vi "Get Subsystem Names.vi"(8 "error in (no error)":errorcluster, 11 "Server URL":refnum<k21>) -> (0 "error out":errorcluster, 2 "Subsystem Names":string[](array[string]), 3 "dup Server URL":refnum<k21>)   [LabVIEW 2024]
doc: "Gets the subsystem names."
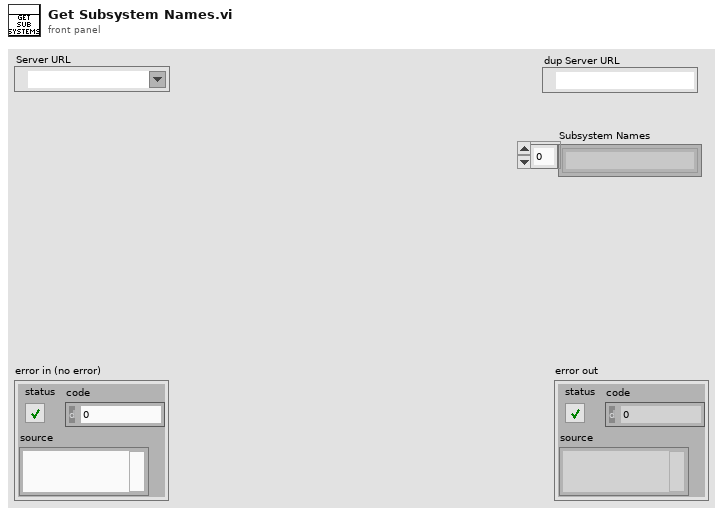
[diagram p1: front panel]
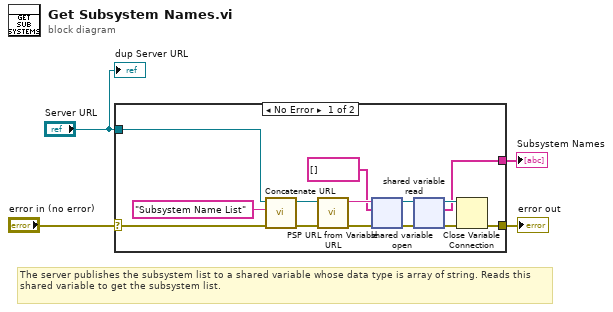
[diagram p0: block diagram]
diagram:
  # "The server publishes the subsystem list to a shared variable whose data type is array of string. Reads this shared variable to get the subsystem list."
  n1 = case shown="No Error" "error in (no error)" {
    selector: "error in (no error)" -> [w18 w19]
    tunnel: [w5 w19] -> w3
    tunnel: "Server URL" -> [w8 _]
    tunnel: [w6 _] -> w1
    frame No Error {
      n2 = call "Concatenate URL.vi"("error in (no error)"=w18, "Child Name"="Subsystem Name List", "Parent URL"=w8) -> ("error out"=w17:errorcluster, "Child URL"=w14:refnum<k21>)  [unwired: 7 in]
      n3 = call "PSP URL from Variable URL.vi"("error in (no error)"=w17, "Shared Variable URL"=w14) -> ("error out"=w16:errorcluster, "PSP URL"=w15:string)  [unwired: 8 in]
      n4 = shared-variable-open(w15, w16, string[] []) -> (w11:refnum<k21>, w12:errorcluster)  [unwired: 1 in]
      n5 = shared-variable-read(w11, w12) -> (w9:refnum<k21>, w10:errorcluster, w6:string[])  [unwired: 1 out]
      n6 = Close Variable Connection(8:w10, 11:w9) -> (0:w5:errorcluster)
    }
    frame Error {
    }
  }
  "error out" <- w3
  "Subsystem Names" <- w1
  "dup Server URL" <- "Server URL"
